vi "Check if Library exists.vi"(8 "error in (no error)":errorcluster, 10 "library name":string, 11 "project ref":refnum<vi>) -> (0 "error out":errorcluster, 3 "found":bool)   [LabVIEW 2021, in "Create Measurement Plug-In Client.lvlib"]
uses:
  Create Measurement Plug-In Client.lvlib
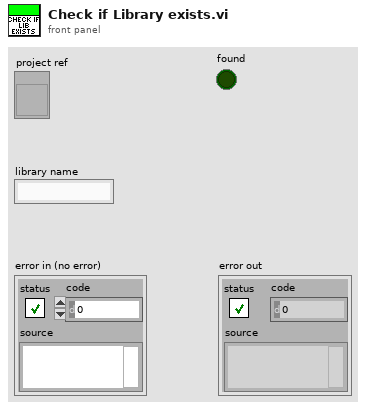
[diagram p1: front panel]
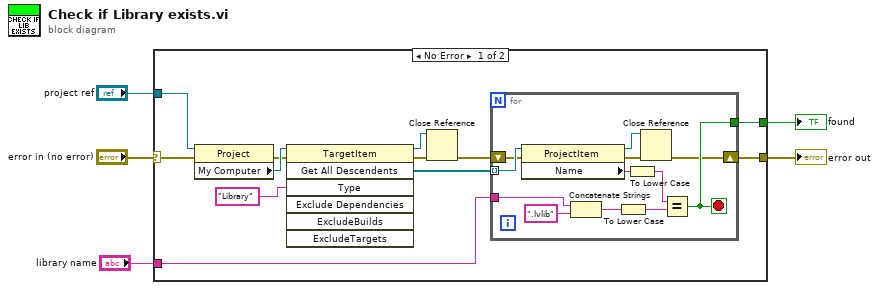
[diagram p0: block diagram]
diagram:
  n1 = case shown="No Error" "error in (no error)" {
    selector: "error in (no error)" -> [w13 w30]
    tunnel: "project ref" -> [w17 _]
    tunnel: "library name" -> [w7 _]
    tunnel: [w12 w30] -> w2
    tunnel: [w6 _] -> w1
    frame No Error {
      n2 = property class="Project"(reference=w17, error in=w13) -> (error out=w15:errorcluster, "My Computer"=w16:refnum<vi>)  [unwired: 1 out]
      n3 = invoke class="TargetItem" method="Get All Descendents"(reference=w16, error in=w15, "Type"="Library") -> (reference out=w10:refnum<vi>, error out=w11:errorcluster, "All Descendents"=w14:refnum<vi>[])  [unwired: 4 in, 4 out]
      n4 = Close Reference(reference=w10, error in (no error)=w11) -> (error out=w9:errorcluster)
      n5 = for {
        tunnel: w14 -> [w29] mode=indexing
        tunnel: w7 -> [w28]
        shift-right: [w19] -> w12
        shift-left: w9 -> [w26]
        tunnel: [w20] -> w6
        stop <- w20 stop-if-true
        n6 = property class="ProjectItem"(reference=w29, error in=w26) -> (reference out=w18:refnum<vi>, error out=w25:errorcluster, "Name"=w22:string)
        n7 = Concatenate Strings(w28, ".lvlib" ("string")) -> (w24:string)
        n8 = To Lower Case(string=w24) -> (all lower case string=w23:string)
        n9 = To Lower Case(string=w22) -> (all lower case string=w21:string)
        n10 = Close Reference(reference=w18, error in (no error)=w25) -> (error out=w19:errorcluster)
        n11 = Equal?(x=w21, y=w23) -> (x = y?=w20:bool)
      }
    }
    frame Error {
    }
  }
  "error out" <- w2
  "found" <- w1
